vi "Close.vi"(8 "error in (no error)":errorcluster, 11 "NI 6514 in":refnum<class "NI 6514.lvclass">) -> (0 "error out":errorcluster, 3 "NI 6514 out":refnum<class "NI 6514.lvclass">)   [LabVIEW 2021, in "Concrete.lvlib" / "NI 6514.lvclass"]
uses:
  NI 6514.lvclass
  NI 6514.lvclass/NI 6514.ctl
  Harware Abstraction/DIO/DIO.lvclass
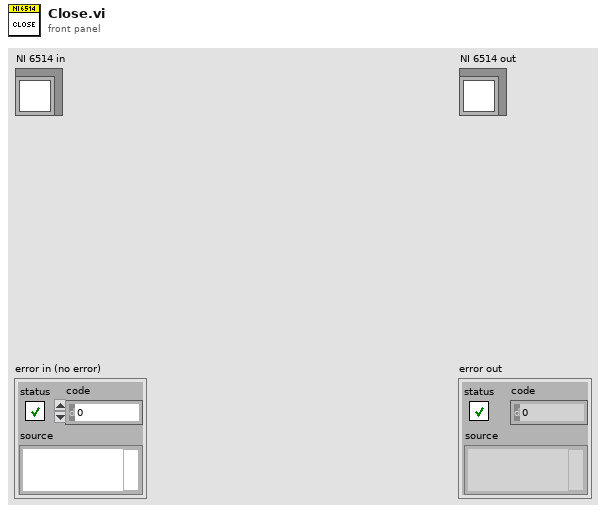
[diagram p1: front panel]
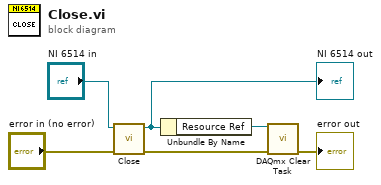
[diagram p0: block diagram]
diagram:
  n1 = call-parent "Close.vi"("error in (no error)"="error in (no error)", "Instrument in"="NI 6514 in") -> ("error out"=w4:errorcluster, "Instrument out"=w2:refnum<class "NI 6514.lvclass">)  [unwired: 8 in]
  "NI 6514 out" <- w2
  n2 = Unbundle By Name(w2) -> ("Resource Ref"=w1:refnum<k21>)
  n3 = call <vilib>:"DAQmx Clear Task.vi"("task in"=w1, "error in"=w4) -> ("error out"=→"error out":errorcluster)  [unwired: 13 in]
